vi "PictureToGreyscaleArrayData.vi"(3 "Bottom":i16, 4 "Right":i16, 5 "Picture":picture) -> (1 "Greyscale Image Data":u8[][](array[numeric]))   [LabVIEW 2020, in "common.lvlib"]
uses:
  common.lvlib
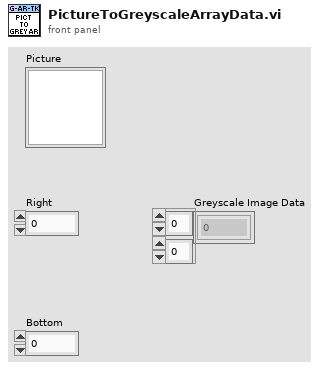
[diagram p1: front panel]
types:
  T1 = cluster{"left":i16, "top":i16, "right":i16, "bottom":i16}
  T2 = typedef "imagedata.ctl" = cluster{"image type":i32, "image depth":i32, "image":u8[], "mask":u8[], "colors":u32[], "Rectangle":cluster{"left":i16, "top":i16, "right":i16, "bottom":i16}}
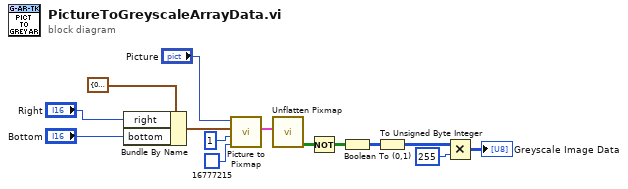
[diagram p0: block diagram]
diagram:
  n1 = Bundle By Name(cluster=T1 {"left"=0, "top"=0, "right"=0, "bottom"=0} ("rect"), "right"="Right", "bottom"="Bottom") -> (w3:T1)
  n2 = call <vilib>:"Picture to Pixmap.vi"("Background Color"=u32 16777215, "depth"=1, "rect"=w3, "picture"="Picture") -> ("image data"=w8:T2)  [unwired: 6 in, 1 out]
  n3 = call <vilib>:"Unflatten Pixmap.vi"("image data"=w8) -> ("1-bit pixmap"=w9:bool[][])  [unwired: 4 in, 6 out]
  n4 = Not(x=w9) -> (.not. x?=w14:bool[][])
  n5 = Boolean To (0,1)(Boolean=w14) -> (0, 1=w10:i16[][])
  n6 = To Unsigned Byte Integer(number=w10) -> (unsigned 8bit integer=w11:u8[][])
  n7 = Multiply(x=w11, y=u8 255) -> (x*y=→"Greyscale Image Data":u8[][])
